vi "testNegativeNumbers.vi"(11 "Test Case In":refnum<class "Test Adder Functionality.lvclass">) -> (0 "error out":errorcluster, 3 "Test Case Out":refnum<class "Test Adder Functionality.lvclass">)   [LabVIEW 2026, in "Test Adder Functionality.lvclass"]
uses:
  Test Adder Functionality.lvclass
  <vilib>/Astemes/LUnit/Test Case.lvclass/Test Case.ctl
  4993e8ee-a06a-463a-9684-69129f64d5ce.vi
  <vilib>/Astemes/LUnit/Core/LUnit Test Case/Private/Append Pass Result.vi
  <vilib>/Astemes/LUnit/Core/LUnit Test Case/Private/Append Fail Result.vi
  4993e8ee-a06a-463a-9684-69129f64d5ce.vi/9c5d11cd-9439-4240-a1ee-d9baace9c924.vi
  <vilib>/Astemes/LUnit/Core/LUnit Test Case/Private/Run In UI.vi
  <vilib>/Utility/error.llb/Clear Errors.vi
  Test Adder Functionality.lvclass/Test Adder Functionality.ctl
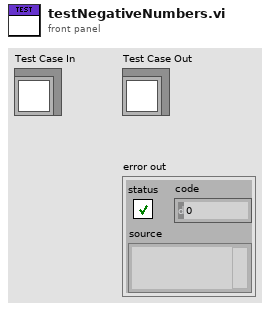
[diagram p1: front panel]
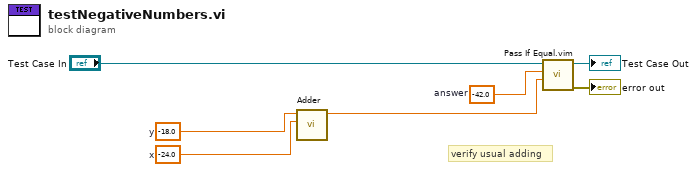
[diagram p0: block diagram]
diagram:
  w1 = -42.0  # answer
  w3 = -24.0  # x
  w4 = -18.0  # y
  # "verify usual adding"
  n1 = call "Adder.vi"("x"=w3, "y"=w4) -> ("x+y"=w2:dbl)  [unwired: 9 in]
  n2 = call "Pass If Equal.vim"("Actual"=w2, "Expected"=w1, "LUnit Test Case In"="Test Case In") -> ("error out"=→"error out":errorcluster, "LUnit Test Case Out"=→"Test Case Out":refnum<class "Test Adder Functionality.lvclass">)  [unwired: 7 in]
